vi "Has Data.vi"(4 "End":dbl, 6 "Start":dbl, 10 "Grouped Channels":T2, 11 "Historian Module in":refnum<class "Historian Module.lvclass">) -> (1 "Has Data":bool, 2 "Needed Data":T1[](array[typedef]), 3 "Historian Module out":refnum<class "Historian Module.lvclass">)   [LabVIEW 2020, in "VolatusHistorian.lvlib" / "Historian Module.lvclass"]
uses:
  Historian Module.lvclass
  Grouped Channels.ctl
  Needed Group Data.ctl
  Historian Module.lvclass/Historian Module.ctl
  Group Buffer DBL/Group Buffer DBL.lvclass/Group Buffer DBL.ctl
  Group Buffer DBL/Check Time Range.vi
  Group Buffer DBL/Group Buffer DBL.lvclass
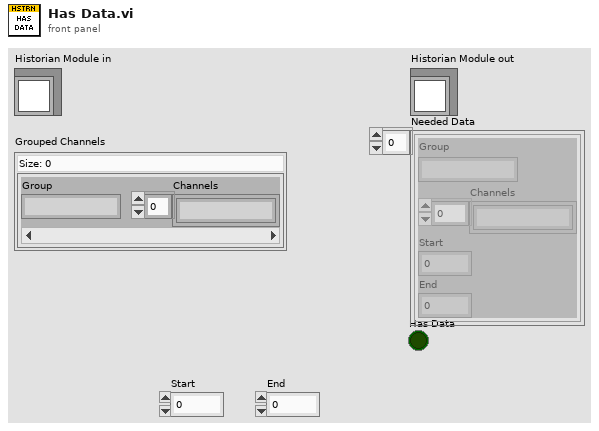
[diagram p1: front panel]
types:
  T1 = typedef "VolatusHistorian.lvlib/Historian Module.lvclass/Needed Group Data.ctl" = cluster{"Group":string, "Channels":string[], "Start":dbl, "End":dbl}
  T2 = typedef "VolatusHistorian.lvlib/Historian Module.lvclass/Grouped Channels.ctl" = map{string, string[]}
  T3 = map{string, refnum<class "Group Buffer DBL.lvclass">}
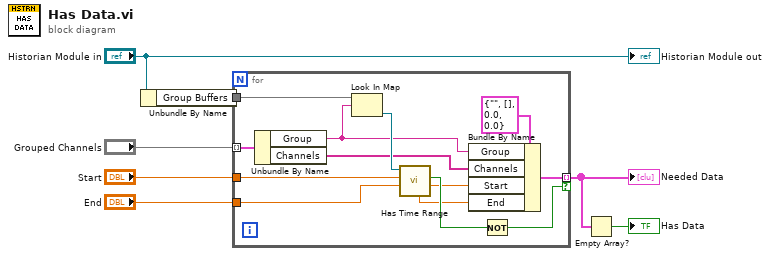
[diagram p0: block diagram]
diagram:
  n1 = Unbundle By Name("Historian Module in") -> ("Group Buffers"=w3:T3)
  n2 = for {
    tunnel: "Grouped Channels" -> [w19] mode=indexing
    tunnel: "Start" -> [w18]
    tunnel: "End" -> [w16]
    tunnel: w3 -> [w20]
    tunnel: [w10] -> w2 mode=indexing if=w9
    n3 = Unbundle By Name(w19) -> ("Group"=w8:string, "Channels"=w13:string[])
    n4 = Look In Map(map=w20, key=w8) -> (value=w17:refnum<class "Group Buffer DBL.lvclass">)  [unwired: 1 in, 1 out]
    n5 = call "Has Time Range.vi"("End"=w16, "Start"=w18, "Group Buffer DBL in"=w17) -> ("Incomplete Start"=w12:dbl, "Complete Range"=w15:bool, "Incomplete End"=w11:dbl)  [unwired: 4 in, 2 out]
    n6 = Bundle By Name(cluster=T1 {"Group"="", "Channels"=[], "Start"=0.0, "End"=0.0} ("Needed Group Data"), "Group"=w8, "Channels"=w13, "Start"=w12, "End"=w11) -> (w10:T1)
    n7 = Not(x=w15) -> (.not. x?=w9:bool)
  }
  "Needed Data" <- w2
  n8 = Empty Array?(array=w2) -> (empty?=→"Has Data":bool)
  "Historian Module out" <- "Historian Module in"
